vi "Finalize.vi"(8 "error in":errorcluster, 11 "Plugin in":refnum<class "FFT.lvclass">) -> (0 "error out":errorcluster, 3 "Plugin out":refnum<class "FFT.lvclass">)   [LabVIEW 2024, in "FFT.lvlib" / "FFT.lvclass"]
uses:
  FFT.lvclass
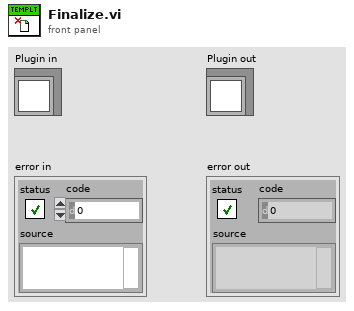
[diagram p1: front panel]
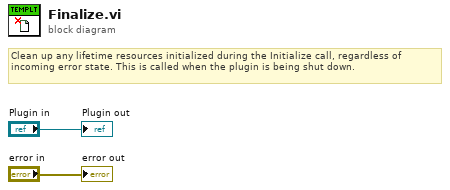
[diagram p0: block diagram]
diagram:
  # "Clean up any lifetime resources initialized during the Initialize call, regardless of incoming error state. This is called when the plugin is being shut down."
  "error out" <- "error in"
  "Plugin out" <- "Plugin in"
